vi "Initialize_Weather_Queues.vi"   [LabVIEW 2013]
uses:
  Globals/Weather_Queues.vi
types:
  T1 = cluster{"Data out":dbl, "Data out":dbl, "Data out":dbl, "Data out":dbl, "Data out":dbl, "Data out":dbl, "Data out":dbl, "Data out":dbl, "Data out":dbl, "Data out":dbl, "Data out":dbl, "Data out":dbl, "Data out":dbl, "Data out":dbl, "seconds since 1Jan1904":dbl}
  T2 = cluster{"Weather data (5s)":refnum<queue>, "Database queue":refnum<queue>, "Message queue":refnum<queue>, "Settings queue":refnum<queue>, "60 mins data queue":refnum<queue>, "48 hrs data queue":refnum<queue>}
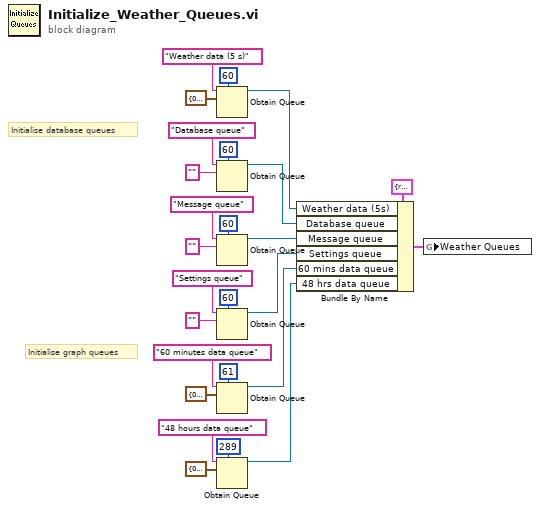
[diagram p0: block diagram]
diagram:
  # "Initialise graph queues"
  # "Initialise database queues"
  n1 = Obtain Queue(max queue size (-1, unlimited)=60, name (unnamed)="Weather data (5 s)", element data type=T1 {"Data out"=0.0, "Data out"=0.0, "Data out"=0.0, "Data out"=0.0, "Data out"=0.0, "Data out"=0.0, "Data out"=0.0, "Data out"=0.0, "Data out"=0.0, "Data out"=0.0, "Data out"=0.0, "Data out"=0.0, "Data out"=0.0, "Data out"=0.0, "seconds since 1Jan1904"=0.0} ("output cluster")) -> (queue out=w7:refnum<queue>)  [unwired: 2 in, 2 out]
  n2 = Obtain Queue(max queue size (-1, unlimited)=60, name (unnamed)="Database queue", element data type="" ("Weather parameter string")) -> (queue out=w6:refnum<queue>)  [unwired: 2 in, 2 out]
  n3 = Obtain Queue(max queue size (-1, unlimited)=60, name (unnamed)="Message queue", element data type="" ("Weather parameter string")) -> (queue out=w2:refnum<queue>)  [unwired: 2 in, 2 out]
  n4 = Obtain Queue(max queue size (-1, unlimited)=60, name (unnamed)="Settings queue", element data type="" ("Weather parameter string")) -> (queue out=w5:refnum<queue>)  [unwired: 2 in, 2 out]
  n5 = Obtain Queue(max queue size (-1, unlimited)=61, name (unnamed)="60 minutes data queue", element data type=T1 {"Data out"=0.0, "Data out"=0.0, "Data out"=0.0, "Data out"=0.0, "Data out"=0.0, "Data out"=0.0, "Data out"=0.0, "Data out"=0.0, "Data out"=0.0, "Data out"=0.0, "Data out"=0.0, "Data out"=0.0, "Data out"=0.0, "Data out"=0.0, "seconds since 1Jan1904"=0.0} ("output cluster")) -> (queue out=w4:refnum<queue>)  [unwired: 2 in, 2 out]
  n6 = Obtain Queue(max queue size (-1, unlimited)=289, name (unnamed)="48 hours data queue", element data type=T1 {"Data out"=0.0, "Data out"=0.0, "Data out"=0.0, "Data out"=0.0, "Data out"=0.0, "Data out"=0.0, "Data out"=0.0, "Data out"=0.0, "Data out"=0.0, "Data out"=0.0, "Data out"=0.0, "Data out"=0.0, "Data out"=0.0, "Data out"=0.0, "seconds since 1Jan1904"=0.0} ("output cluster")) -> (queue out=w3:refnum<queue>)  [unwired: 2 in, 2 out]
  n7 = Bundle By Name(cluster=T2 {"Weather data (5s)"=refnum, "Database queue"=refnum, "Message queue"=refnum, "Settings queue"=refnum, "60 mins data queue"=refnum, "48 hrs data queue"=refnum}, "Weather data (5s)"=w7, "Database queue"=w6, "Message queue"=w2, "Settings queue"=w5, "60 mins data queue"=w4, "48 hrs data queue"=w3) -> (w1:T2)
  n8 = global write "Weather_Queues.vi" "Weather Queues"(w1) -> ()
